vi "Write pre-empt.vi"(8 "error in":errorcluster, 10 "pre-empt":refnum<notifier>, 11 "_Popup in":refnum<class "Popup.lvclass">) -> (0 "error out":errorcluster, 3 "_Popup out":refnum<class "Popup.lvclass">)   [LabVIEW 2021, in "Pop-Up.lvlib" / "Popup.lvclass"]
doc: "write the preemptible notifier\n\n<b>Code Developed By:</b> +\nDaniel Coons +\nhttps://github.com/danielcoons/tsc-pop-up"
uses:
  Popup.lvclass
  Popup.lvclass/Popup.ctl
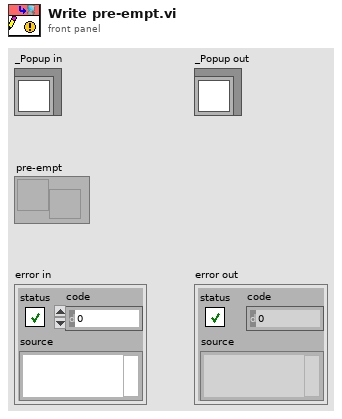
[diagram p1: front panel]
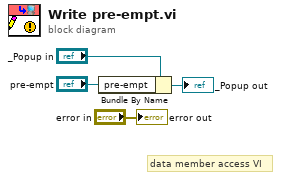
[diagram p0: block diagram]
diagram:
  # "data member access VI"
  n1 = Bundle By Name(cluster="_Popup in", "pre-empt"="pre-empt") -> (→"_Popup out":refnum<class "Popup.lvclass">)
  "error out" <- "error in"
